vi "Verify Font availability.vi"(0 "Font IN":refnum<class "Font Class.lvclass">, 7 "Font name":string, 9 "One button message (F)?":bool, 11 "error in (no error)":errorcluster) -> (4 "Font duplicate":refnum<class "Font Class.lvclass">, 8 "Font":string, 15 "error out":errorcluster)   [LabVIEW 2020, in "Exaprom PDF.lvlib" / "Font Class.lvclass"]
doc: "Version 1.0\nDeveloped by Jean-Marc Simard\nCopyright © 2010, Exaprom Inc.\nAll rights reserved.\nLicense: BSD\n\nWith iTextSharp 4.1.6 (http://itextsharp.sourceforge.net)\nunder Mozilla Public License Version 1.1\n(http://www.mozilla.org/MPL/MPL-1.1.html)"
uses:
  <userlib>/labview-PDF-writer-master/LV Class/Fonts Class/Font Class.lvclass
  <userlib>/labview-PDF-writer-master/LV Class/Fonts Class/Font Class.lvclass/Font Class.ctl
  <userlib>/labview-PDF-writer-master/Exaprom PDF.lvlib
panel:
  out "Font name 2":string
  out "File name":string
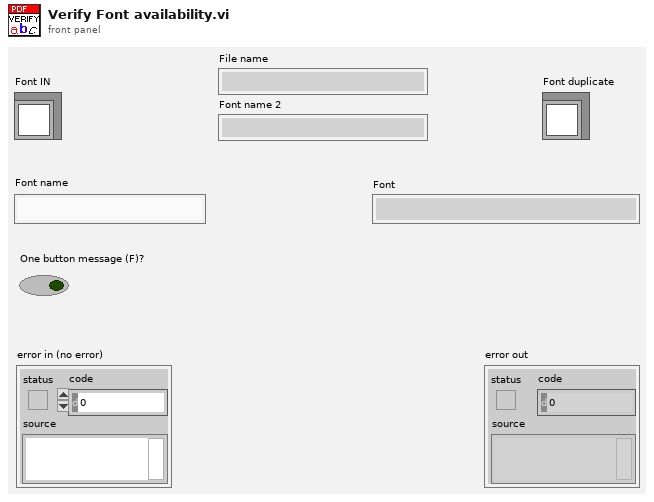
[diagram p1: front panel]
types:
  T1 = cluster{"Font name":string, "File name":string}[]
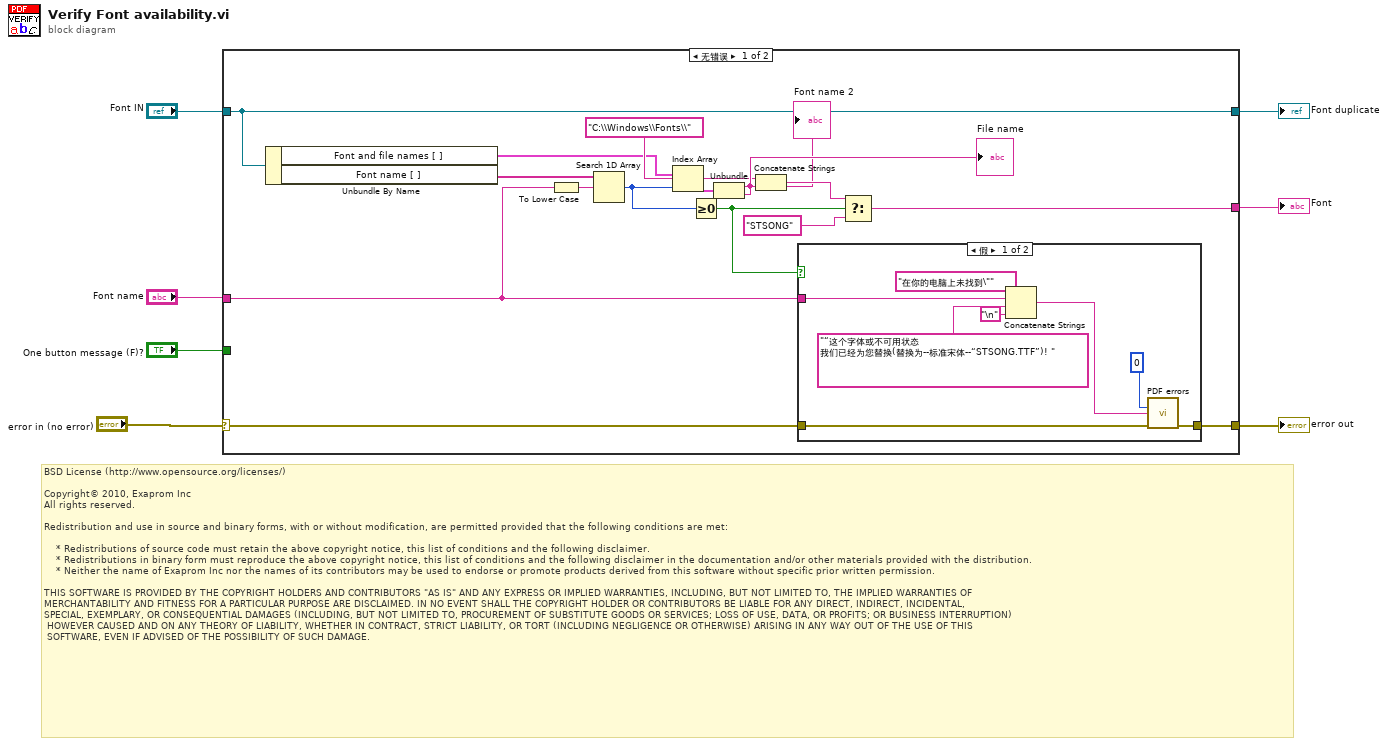
[diagram p0: block diagram]
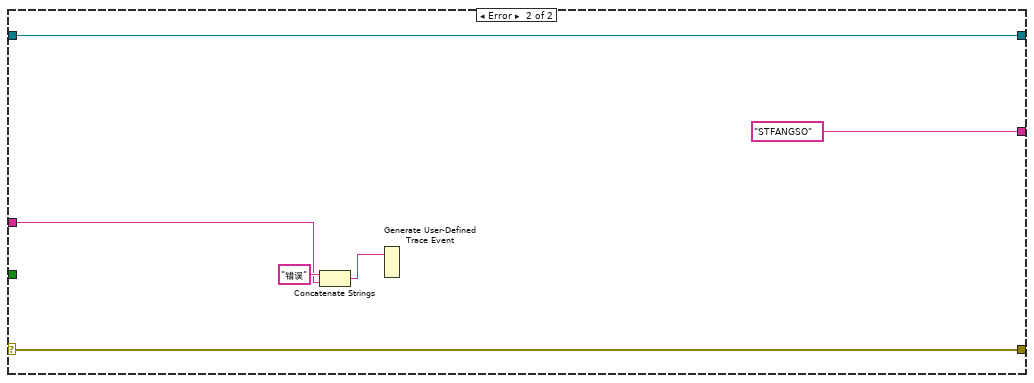
[diagram p3: hidden frame]
diagram:
  # "BSD License (http://www.opensource.org/licenses/)\n\nCopyright© 2010, Exaprom Inc\nAll rights reserved.\n\nRedistribution and use in source and binary forms, with or without modification, are permitted provided that the following conditions are met:\n\n    * Redistributions of source code must retain the above copyright notice, this list of conditions and the following disclaimer.\n    * Redistributions in binary form must reproduce the above copyright notice, this list of conditions and the following disclaimer in the documentation and/or other materials provided with the distribution.\n    * Neither the name of Exaprom Inc nor the names of its contributors may be used to endorse or promote products derived from this software without specific prior written permission.\n\nTHIS SOFTWARE IS PROVIDED BY THE COPYRIGHT HOLDERS AND CONTRIBUTORS \"AS IS\" AND ANY EXPRESS OR IMPLIED WARRANTIES, INCLUDING, BUT NOT LIMITED TO, THE IMPLIED WARRANTIES OF \nMERCHANTABILITY AND FITNESS FOR A PARTICULAR PURPOSE ARE DISCLAIMED. IN NO EVENT SHALL THE COPYRIGHT HOLDER OR CONTRIBUTORS BE LIABLE FOR ANY DIRECT, INDIRECT, INCIDENTAL,\nSPECIAL, EXEMPLARY, OR CONSEQUENTIAL DAMAGES (INCLUDING, BUT NOT LIMITED TO, PROCUREMENT OF SUBSTITUTE GOODS OR SERVICES; LOSS OF USE, DATA, OR PROFITS; OR BUSINESS INTERRUPTION)\n HOWEVER CAUSED AND ON ANY THEORY OF LIABILITY, WHETHER IN CONTRACT, STRICT LIABILITY, OR TORT (INCLUDING NEGLIGENCE OR OTHERWISE) ARISING IN ANY WAY OUT OF THE USE OF THIS\n SOFTWARE, EVEN IF ADVISED OF THE POSSIBILITY OF SUCH DAMAGE."
  n1 = case shown="无错误" "error in (no error)" {
    selector: "error in (no error)" -> [w13 w38]
    tunnel: [w14 w38] -> w7
    tunnel: [w16 "STFANGSO"] -> w5
    tunnel: "Font name" -> [w8 w33]
    tunnel: "One button message (F)?" -> [_ _]
    tunnel: "Font IN" -> [w10 w36]
    tunnel: [w10 w36] -> w1
    frame No Error {
      n2 = Unbundle By Name(w10) -> ("Font and file names [ ]"=w12:T1, "Font name [ ]"=w11:string[])
      n3 = To Lower Case(string=w8) -> (all lower case string=w23:string)
      n4 = Search 1D Array(1D array=w11, element=w23) -> (index of element=w20:i32)  [unwired: 1 out]
      n5 = Index Array(array=w12, index=w20) -> (element=w18:cluster{"Font name":string, "File name":string})
      n6 = Greater Or Equal To 0?(x=w20) -> (x >= 0?=w15:bool)
      n7 = Unbundle(w18) -> ("Font name"=→"Font name 2":string, "File name"=w19:string)
      "File name" <- w19
      n8 = Concatenate Strings("C:\\Windows\\Fonts\\", w19) -> (w21:string)
      n9 = case shown="假" w15 {
        tunnel: w8 -> [w30 _]
        tunnel: [w27 w32] -> w14
        tunnel: w13 -> [w26 w32]
        frame False {
          n10 = Concatenate Strings("在你的电脑上未找到\"", w30, "“这个字体或不可用状态 我们已经为您替换(替换为--标准宋体--“STSONG.TTF”)! " ("string"), "\n") -> (w25:string)
          n11 = call <userlib>:"PDF errors.vi"("code"=0, "Additionnal information"=w25, "error in (no error)"=w26) -> ("error out"=w27:errorcluster)  [unwired: 12 out]
        }
        frame True {
        }
      }
      n12 = Select(t=w21, s=w15, f="STSONG") -> (s? t:f=w16:string)
    }
    frame Error {
      n13 = Concatenate Strings("错误" ("字符串"), w33) -> (w34:string)
      n14 = Generate User-Defined Trace Event(2:w34) -> ()  [unwired: 1 in]
    }
  }
  "error out" <- w7
  "Font" <- w5
  "Font duplicate" <- w1
